vi "startSerial.vi"(8 "error in (no error)":errorcluster, 11 "FlukeDMM in":refnum<class "FlukeDMM.lvclass">) -> (0 "error out":errorcluster, 3 "FlukeDMM out":refnum<class "FlukeDMM.lvclass">)   [LabVIEW 2013, in "FlukeDMM.lvlib" / "FlukeDMM.lvclass"]
uses:
  <userlib>/Common/Devices/FlukeDMM/FlukeDMM/FlukeDMM.lvclass
  <userlib>/Common/Devices/FlukeDMM/FlukeDMM/FlukeDMM.lvclass/FlukeDMM.ctl
  <userlib>/Common/SerialProtocols/SerialCommunicator/SerialCommunicator.lvclass
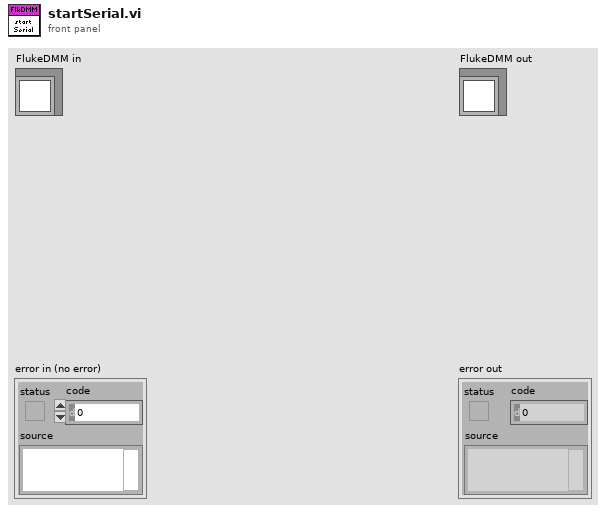
[diagram p1: front panel]
types:
  T1 = typedef "SerialProtocols.lvlib/SerialConfig.ctl" = cluster{"Serial Protocol":T2, "Protocol Parameters":T3, "Serial Message Parameters":T4}
  T2 = typedef "SerialProtocols.lvlib/SerialProtocol.ctl" = enum16{"RS232", "RS485", "SerialSimulator"}
  T3 = typedef "SerialProtocols.lvlib/ProtocolParameters.ctl" = cluster{"VISA resource name":refnum<visa-resource-name>, "Baud Rate":u32, "Data Bits":u16, "Parity":enum16{"None", "Odd", "Even", "Mark", "Space"}, "Flow Control":u16, "Stop Bits":u16, "Timeout (ms)":u32}
  T4 = typedef "SerialProtocols.lvlib/SerialMessageParameters.ctl" = cluster{"Byte Count":u32, "Enable Termination Character":bool, "Termination Char":u8}
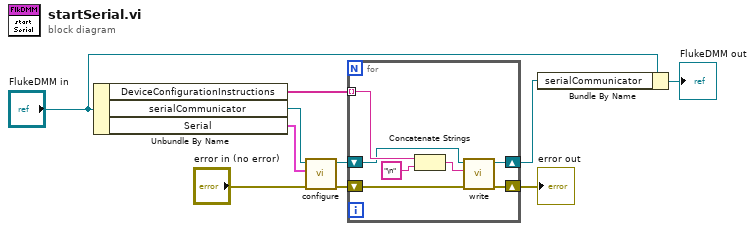
[diagram p0: block diagram]
diagram:
  n1 = Unbundle By Name("FlukeDMM in") -> ("DeviceConfigurationInstructions"=w1:string[], "serialCommunicator"=w9:refnum<class "SerialCommunicator.lvclass">, "Serial"=w10:T1)
  n2 = call-dynamic "configure.vi"("error in (no error)"="error in (no error)", "SerialConfig"=w10, "SerialCommunicator in"=w9) -> ("error out"=w4:errorcluster, "SerialCommunicator out"=w5:refnum<class "SerialCommunicator.lvclass">)  [unwired: 7 in]
  n3 = for {
    tunnel: w1 -> [w17] mode=indexing
    shift-right: [w14] -> w3
    shift-left: w5 -> [w15]
    shift-right: [w11] -> w2
    shift-left: w4 -> [w12]
    n4 = Concatenate Strings(w17, "\n" ("string")) -> (w13:string)
    n5 = call-dynamic "write.vi"("error in (no error)"=w12, "writeString"=w13, "SerialCommunicator in"=w15) -> ("error out"=w11:errorcluster, "SerialCommunicator out"=w14:refnum<class "SerialCommunicator.lvclass">)  [unwired: 7 in]
  }
  "error out" <- w2
  n6 = Bundle By Name(cluster="FlukeDMM in", "serialCommunicator"=w3) -> (→"FlukeDMM out":refnum<class "FlukeDMM.lvclass">)
